vi "HIOKI PW3390 Conf Timer.vi"(0 "VISA Resource":refnum<visa-resource-name>, 1 "Set/Query (F: Set)":bool, 5 "Mode (0: OFF)":enum16{"OFF", "ON"}(ring), 7 "Time (0:01:00)":cluster{"Hour":i32, "Minute":i32, "Second":i32}={"Hour"=0, "Minute"=1, "Second"=0} {"Second" min=0 max=59; "Minute" min=0 max=59; "Hour" min=0 max=9999}, 11 "error in (no error)":errorcluster, 12 "OPC query (T: ON)":bool=TRUE, 13 "Error Out (F: Off)":bool) -> (4 "VISA Resource out":refnum<visa-resource-name>, 6 "Mode out":enum16{"OFF", "ON"}(ring), 8 "Time out":cluster{"Hour":i32, "Minute":i32, "Second":i32}={"Hour"=0, "Minute"=1, "Second"=0}, 15 "error out":errorcluster)   [LabVIEW 2009]
doc: "Set/Query\n Set: Send the setting commands for the device.\n Query: Query the setting of the device.\n\nMode\n Sets the ON/OFF of the Timer Control.\n\nTime\n Sets the Timer Control in hours, minutes and seconds.\n<B>Note</B>\nThe timer range setting is from 10 seconds to 9999 hours \n59 minutes 59 seconds."
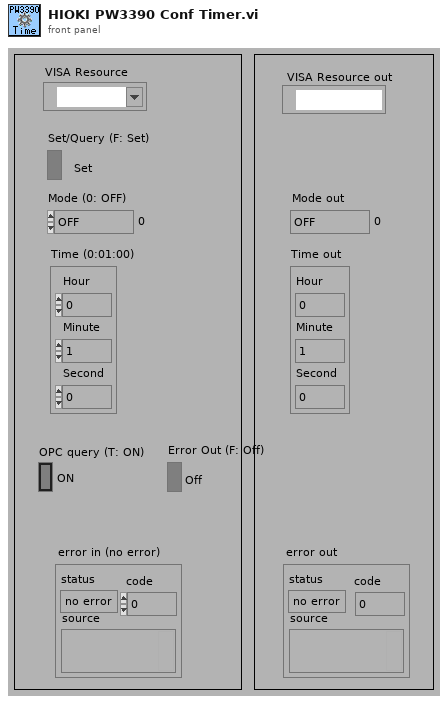
[diagram p1: front panel]
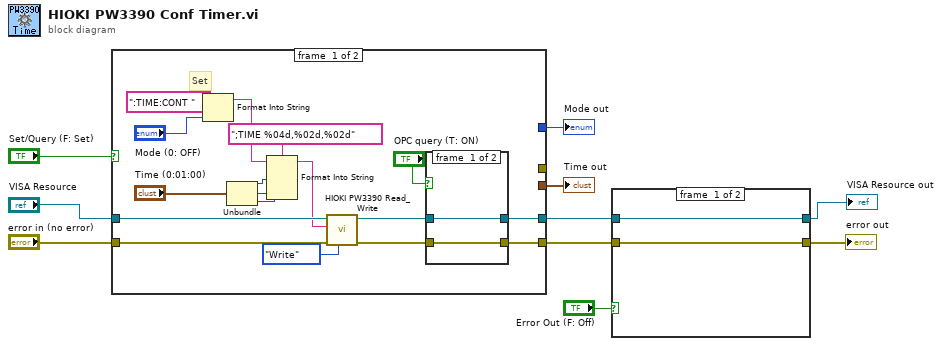
[diagram p0: block diagram]
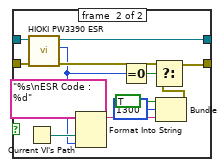
[diagram p2: hidden frame]
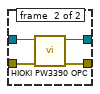
[diagram p3: hidden frame]
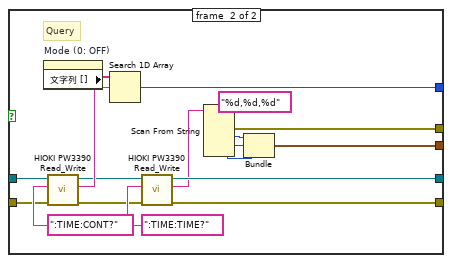
[diagram p4: hidden frame]
diagram:
  n1 = case shown="FALSE" "Set/Query (F: Set)" {
    tunnel: "error in (no error)" -> [w26 w50]
    tunnel: [w11 w42] -> w7
    tunnel: "VISA Resource" -> [w27 w49]
    tunnel: [w12 w41] -> w6
    tunnel: [_ w47] -> w4
    tunnel: [_ w36] -> w3
    tunnel: [_ w34] -> _
    frame #0 {
      # "Set"
      n2 = Format Into String(initial string=":TIME:CONT ", "Mode (0: OFF)") -> (resulting string=w16:string)  [unwired: 2 in, 1 out]
      n3 = Unbundle("Time (0:01:00)") -> ("Hour"=w22:i32, "Minute"=w20:i32, "Second"=w19:i32)
      n4 = Format Into String(format string=";TIME %04d,%02d,%02d", initial string=w16, w22, w20, w19) -> (resulting string=w17:string)  [unwired: 1 in, 1 out]
      n5 = call <instrlib>:"HIOKI PW3390 Read_Write.vi"("Read/Write"=enum16{"Read", "Write"}."Write", "error in (no error)"=w26, "data in"=w17, "VISA Resource"=w27) -> ("error out"=w13:errorcluster, "VISA Resource out"=w14:refnum<visa-resource-name>)  [unwired: 5 in, 1 out]
      n6 = case shown="TRUE" "OPC query (T: ON)" {
        tunnel: [w29 w33] -> w12
        tunnel: [w28 w32] -> w11
        tunnel: w14 -> [w29 w31]
        tunnel: w13 -> [w28 w30]
        frame #0 {
        }
        frame #1 {
          n7 = call <instrlib>:"HIOKI PW3390 OPC.vi"("error in (no error)"=w30, "VISA Resource"=w31) -> ("error out"=w32:errorcluster, "VISA Resource out"=w33:refnum<visa-resource-name>)  [unwired: 7 in, 1 out]
        }
      }
    }
    frame #1 {
      # "Query"
      n8 = property on="Mode (0: OFF)" class="Enum (strict)"() -> ("文字列 []"=w46:string[])  [unwired: 2 in, 2 out]
      n9 = call <instrlib>:"HIOKI PW3390 Read_Write.vi"("error in (no error)"=w50, "data in"=":TIME:CONT?", "VISA Resource"=w49) -> ("error out"=w43:errorcluster, "data out"=w48:string, "VISA Resource out"=w44:refnum<visa-resource-name>)  [unwired: 6 in]
      n10 = Search 1D Array(1D array=w46, element=w48) -> (index of element=w47:i32)  [unwired: 1 in]
      n11 = call <instrlib>:"HIOKI PW3390 Read_Write.vi"("error in (no error)"=w43, "data in"=":TIME:TIME?", "VISA Resource"=w44) -> ("error out"=w42:errorcluster, "data out"=w40:string, "VISA Resource out"=w41:refnum<visa-resource-name>)  [unwired: 6 in]
      n12 = Scan From String(format string="%d,%d,%d" ("形式文字列"), input string=w40) -> (error out=w34:errorcluster, output 1=w39:i32, output 2=w38:i32, output 3=w37:i32)  [unwired: 5 in, 2 out]
      n13 = Bundle(w39, w38, w37) -> (w36:cluster{i32, i32, i32})  [unwired: 1 in]
    }
  }
  "Mode out" <- w4
  "Time out" <- w3
  n14 = case shown="TRUE" "Error Out (F: Off)" {
    tunnel: w6 -> [w53 w66]
    tunnel: w7 -> [w52 w65]
    tunnel: [w52 w55] -> w5
    tunnel: [w53 w64] -> w1
    frame #0 {
    }
    frame #1 {
      n15 = Current VI's Path() -> (path=w62:path)
      n16 = call <instrlib>:"HIOKI PW3390 ESR.vi"("error in (no error)"=w65, "VISA Resource"=w66) -> ("error out"=w56:errorcluster, "Output Value"=w54:u8, "VISA Resource out"=w64:refnum<visa-resource-name>)  [unwired: 6 in, 1 out]
      n17 = Format Into String(format string="%s\nESR Code : %d", w62, w54) -> (resulting string=w58:string)  [unwired: 2 in, 1 out]
      n18 = Equal To 0?(x=w54) -> (x = 0?=w63:bool)
      n19 = Bundle("status"=TRUE, "code"=1300, w58) -> (w57:cluster{"status":bool, "code":i32, string})  [unwired: 1 in]
      n20 = Select(t=w56, s=w63, f=w57) -> (s? t:f=w55:errorcluster)
    }
  }
  "error out" <- w5
  "VISA Resource out" <- w1
